vi "GOLPI simple testing.vi"() -> ()   [LabVIEW 2020, in "GOLPI library.lvlib"]
uses:
  GOLPI library.lvlib
  Get String.vi
  Get Double.vi
  Get Double Complex.vi
  Get 1D Array String.vi
  Get 1D Array Double.vi
  Get 1D Array Double Complex.vi
  Get 2D Array Double.vi
  Get 2D Array Double Complex.vi
panel:
  in  "wait for exit\n(press this again to exit)":bool=TRUE
  in  "Bitstream":bool
  in  "hide debug console":bool
  in  "data type array 5":cdb[][](array[numeric])
  in  "data type array 4":dbl[][](array[numeric])
  in  "use temporary file?":bool
  in  "data type array 3":cdb[](array[numeric])
  in  "data type array 2":string[](array[string])
  in  "data type 4":cdb
  in  "data type 3":dbl
  in  "Get variable":T1(tab)=enum."vector reals"
  out "s":string
  out "r":dbl format="%.2f"
  out "c":cdb format="%.2f"
  out "vs length":i32
  out "vs":string[](array[string])
  out "vr":dbl[](array[numeric])
  out "vr length":i32
  out "vc length":i32
  out "vc":cdb[](array[numeric])
  out "mr":dbl[][](array[numeric]) format="%.2f"
  out "mr sizes":i32[](array[numeric])
  out "mc sizes":i32[](array[numeric])
  out "mc":cdb[][](array[numeric]) format="%.2f"
  in  "data type array":dbl[](array[numeric])
  in  "data type":string
  in  "variable name":string="x"
  in  "command":string="x=[1 2 3]\ndisp('OK')"
  out "GNU Octave version":string
  out "exit code":i32
  out "error out":errorcluster
  out "read buffer":string
  in  "Octave binary directory":path=path "C:/Program Files/Octave-3.6.2/bin"
  in  "Working directory":path=path "C:/"
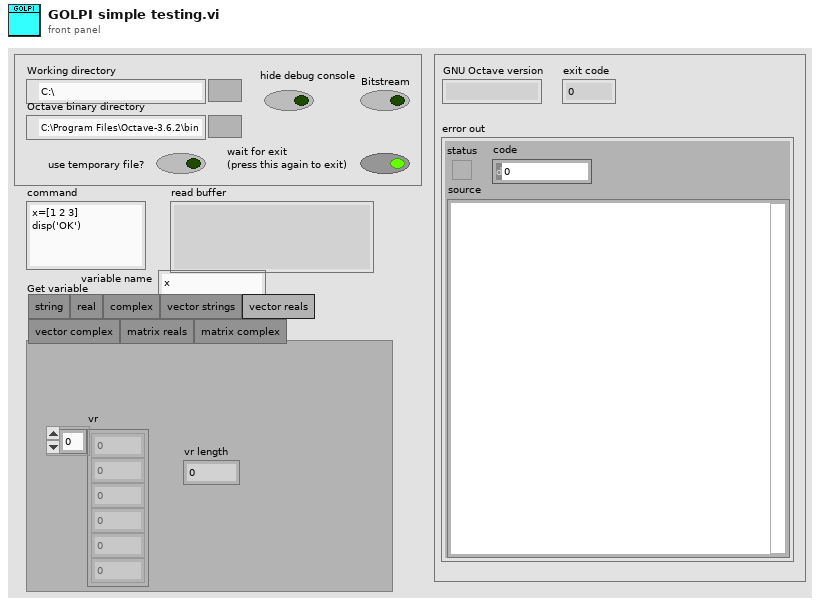
[diagram p1: front panel]
types:
  T1 = enum32{"string", "real", "complex", "vector strings", "vector reals", "vector complex", "matrix reals", "matrix complex"}
  T2 = typedef "GOLPI library.lvlib/GOLPI reference Type Def.ctl" = cluster{"pipe handle":T3, "fast read timeout [ms]":u32, "fast read settle time [ms]":u32, "fast read to multiple [ms]":u32, "max elements per input line":u32, "slow read timeout [ms]":u32, "stdin double format specifier":string, "max elements per stdout output column":u32, "console mode bitstream":bool, "bitstream first read timeout [ms]":u32, "bitstream read timeout [ms]":u32, "struct transfer possible":bool, "matlab mode":bool}
  T3 = typedef "LV Process library.lvlib/Pipe Handle.ctl" = cluster{"lv_proc.dll file path":path, "process instance handle":u32[], "debug mode":bool, "debug data":cluster{"time":timestamp, "stdin":bool, "data":string}[]}
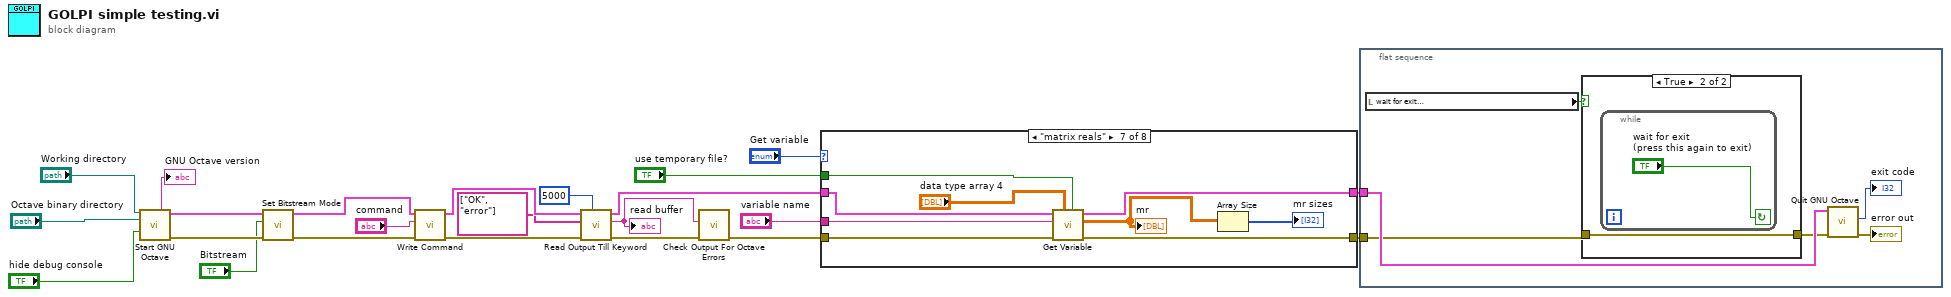
[diagram p0: block diagram]
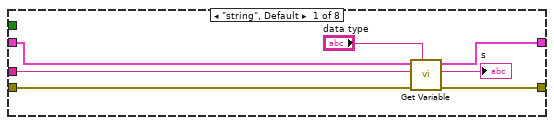
[diagram p3: hidden frame]
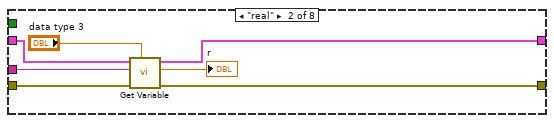
[diagram p4: hidden frame]
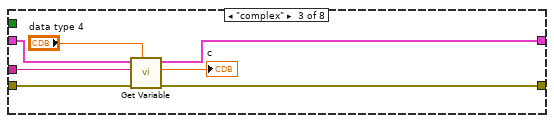
[diagram p5: hidden frame]
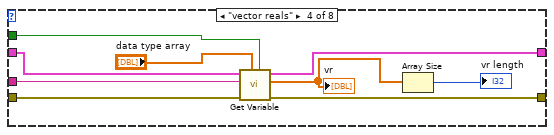
[diagram p6: hidden frame]
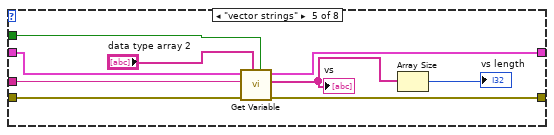
[diagram p7: hidden frame]
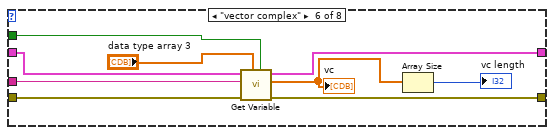
[diagram p8: hidden frame]
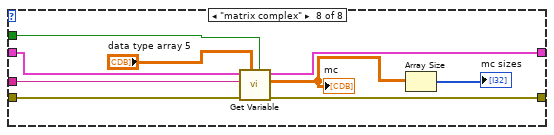
[diagram p9: hidden frame]
diagram:
  n1 = call "Start GNU Octave.vi"("working dir (user home)"="Working directory", "octave binary file or dir (autofind)"="Octave binary directory", "hide debug console (T)"="hide debug console") -> ("GNU Octave version"=→"GNU Octave version":string, "GOLPI ref. out"=w4:T2, "error out"=w6:errorcluster)  [unwired: 9 in, 1 out]
  n2 = call "Set Bitstream Mode.vi"("error in"=w6, "Bitstream mode (F)"="Bitstream", "GOLPI ref. in"=w4) -> ("error out"=w5:errorcluster, "GOLPI ref. out"=w3:T2)  [unwired: 7 in]
  n3 = call "Write Command.vi"("error in"=w5, "command"="command", "GOLPI ref. in"=w3) -> ("error out"=w20:errorcluster, "GOLPI ref. out"=w21:T2)  [unwired: 7 in]
  n4 = call "Read Output Till Keyword.vi"("timeout [ms]"=u32 5000, "error in"=w20, "keywords"=string[] ["OK", "error"], "GOLPI ref. in"=w21) -> ("error out"=w16:errorcluster, "read buffer"=w14:string, "GOLPI ref. out"=w19:T2)  [unwired: 4 in, 1 out]
  "read buffer" <- w14
  n5 = call "Check Output For Octave Errors.vi"("error in"=w16, "read buffer"=w14) -> ("error out"=w15:errorcluster)  [unwired: 9 in]
  n6 = case shown="\"matrix reals\"" "Get variable" {
    tunnel: w19 -> [w29 w34 w42 w51 w59 w67 w80 w88]
    tunnel: [w26 w32 w39 w50 w56 w64 w76 w85] -> w18
    tunnel: [w27 w31 w38 w49 w57 w65 w77 w84] -> w1
    tunnel: "variable name" -> [w24 w35 w40 w52 w60 w68 w79 w86]
    tunnel: w15 -> [w28 w36 w41 w53 w58 w66 w78 w87]
    tunnel: "use temporary file?" -> [_ _ _ w46 w54 w63 w75 w83]
    frame "string", Default {
      n7 = call-poly "Get Variable.vi"("data type of variable"="data type", "error in"=w28, "variable name"=w24, "GOLPI ref. in"=w29) -> ("error out"=w27:errorcluster, "value"=→"s":string, "GOLPI ref. out"=w26:T2)  [unwired: 5 in]
    }
    frame "real" {
      n8 = call-poly "Get Variable.vi"("data type of variable"="data type 3", "error in"=w36, "variable name"=w35, "GOLPI ref. in"=w34) -> ("error out"=w31:errorcluster, "value"=→"r":dbl, "GOLPI ref. out"=w32:T2)  [unwired: 5 in]
    }
    frame "complex" {
      n9 = call-poly "Get Variable.vi"("data type of variable"="data type 4", "error in"=w41, "variable name"=w40, "GOLPI ref. in"=w42) -> ("error out"=w38:errorcluster, "value"=→"c":cdb, "GOLPI ref. out"=w39:T2)  [unwired: 5 in]
    }
    frame "vector reals" {
      n10 = call-poly "Get Variable.vi"("use temporary file? (F)"=w46, "data type of variable"="data type array", "error in"=w53, "variable name"=w52, "GOLPI ref. in"=w51) -> ("error out"=w49:errorcluster, "value"=w45:dbl[], "GOLPI ref. out"=w50:T2)  [unwired: 4 in]
      "vr" <- w45
      n11 = Array Size(array=w45) -> (size(s)=→"vr length":i32)
    }
    frame "vector strings" {
      n12 = call-poly "Get Variable.vi"("use temporary file? (F)"=w54, "data type of variable"="data type array 2", "error in"=w58, "variable name"=w60, "GOLPI ref. in"=w59) -> ("error out"=w57:errorcluster, "value"=w55:string[], "GOLPI ref. out"=w56:T2)  [unwired: 4 in]
      "vs" <- w55
      n13 = Array Size(array=w55) -> (size(s)=→"vs length":i32)
    }
    frame "vector complex" {
      n14 = call-poly "Get Variable.vi"("use temporary file? (F)"=w63, "data type of variable"="data type array 3", "error in"=w66, "variable name"=w68, "GOLPI ref. in"=w67) -> ("error out"=w65:errorcluster, "value"=w69:cdb[], "GOLPI ref. out"=w64:T2)  [unwired: 4 in]
      "vc" <- w69
      n15 = Array Size(array=w69) -> (size(s)=→"vc length":i32)
    }
    frame "matrix reals" {
      n16 = call-poly "Get Variable.vi"("use temporary file? (F)"=w75, "data type of variable"="data type array 4", "error in"=w78, "variable name"=w79, "GOLPI ref. in"=w80) -> ("error out"=w77:errorcluster, "value"=w72:dbl[][], "GOLPI ref. out"=w76:T2)  [unwired: 4 in]
      "mr" <- w72
      n17 = Array Size(array=w72) -> (size(s)=→"mr sizes":i32[])
    }
    frame "matrix complex" {
      n18 = call-poly "Get Variable.vi"("use temporary file? (F)"=w83, "data type of variable"="data type array 5", "error in"=w87, "variable name"=w86, "GOLPI ref. in"=w88) -> ("error out"=w84:errorcluster, "value"=w81:cdb[][], "GOLPI ref. out"=w85:T2)  [unwired: 4 in]
      "mc" <- w81
      n19 = Array Size(array=w81) -> (size(s)=→"mc sizes":i32[])
    }
  }
  n20 = flat-sequence {
    tunnel: w18 -> [w93]
    tunnel: w1 -> [w91]
    frame #0 {
      n21 = local read "wait for exit\n(press this again to exit)"() -> (w92:bool)
      n22 = case shown="True" w92 {
        tunnel: [w96 w97] -> w90
        tunnel: w91 -> [w96 w97]
        frame False {
        }
        frame True {
          n23 = while {
            stop <- "wait for exit\n(press this again to exit)" continue-if-true
          }
        }
      }
      n24 = call "Quit GNU Octave.vi"("error in"=w90, "GOLPI ref. in"=w93) -> ("error out"=→"error out":errorcluster, "exit code"=→"exit code":i32)  [unwired: 8 in]
    }
  }
